vi "Dequeue.vi"(8 "ErrorArray":errorcluster[](array[cluster])) -> (0 "ErrorArray":errorcluster[](array[cluster]), 1 "Data":variant, 2 "Msg":string)   [LabVIEW 2014, in "Framework.lvlib"]
uses:
  Framework.lvlib
  Typedef/MsgQueue.ctl
  <userlib>/NIST/NISTErrorLib/NISTErrorLib.lvlib
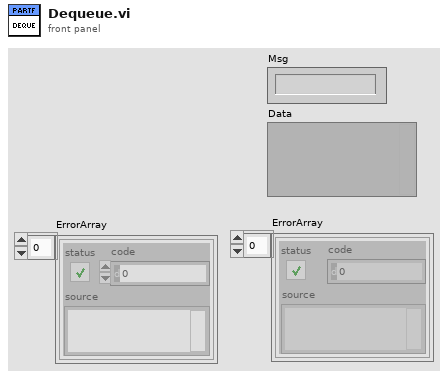
[diagram p1: front panel]
types:
  T1 = typedef "Framework.lvlib/MsgQueue.ctl" = cluster{"Msg":string, "Data":variant}
  T2 = typedef "Framework.lvlib/QueRef.ctl" = refnum<queue>
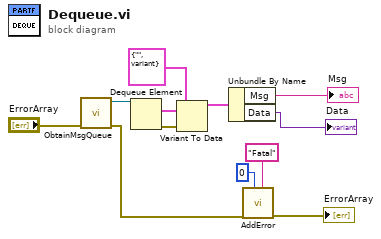
[diagram p0: block diagram]
diagram:
  n1 = call "ObtainMsgQueue.vi"("ErrorArray"="ErrorArray") -> ("ErrorArray"=w10:errorcluster[], "QueRef"=w11:T2)  [unwired: 9 in]
  n2 = Dequeue Element(queue=w11) -> (element=w7:T1, error out=w6:errorcluster)  [unwired: 2 in, 2 out]
  n3 = Variant To Data(error in=w6, type=T1 {"Msg"="", "Data"=variant} ("MsgQueue"), Variant=w7) -> (data=w4:T1)  [unwired: 1 out]
  n4 = Unbundle By Name(w4) -> ("Msg"=→"Msg":string, "Data"=→"Data":variant)
  n5 = call <userlib>:"AddError.vi"("Severity"="Fatal", "Priority"=u8 0, "ErrorArray"=w10) -> ("ErrorArray"=→"ErrorArray":errorcluster[])  [unwired: 7 in, 1 out]
